vi "SP Format CH Plot.vi"(0 "CH Control":T19={"Trace On"=TRUE, "Measure"=0, "Format"=0, "Autoscale"=TRUE, "Reference"=0.0, "\nRefUnit"="dB/Div", "Position"=5.0, "Scale"=10.0, "ScaleUnit"="dB/Div", "LimitOn"=TRUE, "LimitFill"=FALSE, "Display Data"=0, "Show Markers"=TRUE, "SXX"=""} {"Measure" items=["S11", "S21", "S12", "S22"]; "Reference" format="%#.2g"; "Display Data" items=["Data", "Memory", "Data/Memory"]; "Format" items=["Log Mag", "Phase", "Expanded Phase", "Delay", "Smith", "Polar", "Lin Mag", "SWR", "Loss", "Real", "Imaginary"]; "Scale" min=0.001 step=1.0 format="%#.2g"; "Position" min=0.0 max=10.0}, 1 "Results":waveform(dbl)[](array[waveform]), 2 "Limits":T16[](array[typedef]) {"Parameter"."Stimulus Port" min=1 step=1; "Parameter"."Response Port" min=1 step=1}, 3 "Filter Limits":T1[](array[typedef]) {"Parameter"."Stimulus Port" min=1 step=1; "Parameter"."Response Port" min=1 step=1; "Passband"."Bandwidth Attn" format="%.3g"; "Passband"."Stop/Span" format="%.3g"; "Passband"."Start/Center" format="%.3g"}, 5 "Frequency Attributes":cluster{"F0":dbl, "dF":dbl}, 9 "Formatted Data":bool, 11 "error in (no error)":errorcluster, 12 "Units":T13, 13 "Frequency (MHz) In":cluster{"Start":dbl, "Stop":dbl}) -> (4 "X-Y Plot":cluster{"X":dbl[], "Y":dbl[]}[](array[cluster]), 6 "Frequency (MHz) Out":cluster{"Start":dbl, "Stop":dbl}, 10 "Limit Traces":T15, 15 "error out":errorcluster)   [LabVIEW 2011]
uses:
  TypeDefs/SP Display Trace Controls.ctl
  TypeDefs/SP Display Format.ctl
  TypeDefs/SP Display Data.ctl
  TypeDefs/SP Limit.ctl
  TypeDefs/SP Parameter.ctl
  TypeDefs/SP Format.ctl
  TypeDefs/SP Limit Type.ctl
  TypeDefs/SP Limit Point.ctl
  Test Referential Limit.ctl
  TypeDefs/SP Frequency Units.ctl
  TypeDefs/SP Filter.ctl
  TypeDefs/SP Filter Type.ctl
  TypeDefs/SP Filter Passband.ctl
  TypeDefs/SP Frequency Format.ctl
  TypeDefs/SP Filter Ripple.ctl
  TypeDefs/SP Attenuation Point.ctl
  TypeDefs/SP Attenuation Type.ctl
  TypeDefs/SP Skirt Rejection Point.ctl
  TypeDefs/SP Relative Loss.ctl
panel:
  out "Waveform Plot":cluster{"x0":dbl, "dx":dbl, "Y":dbl[]}[](array[cluster])
  # "Div"
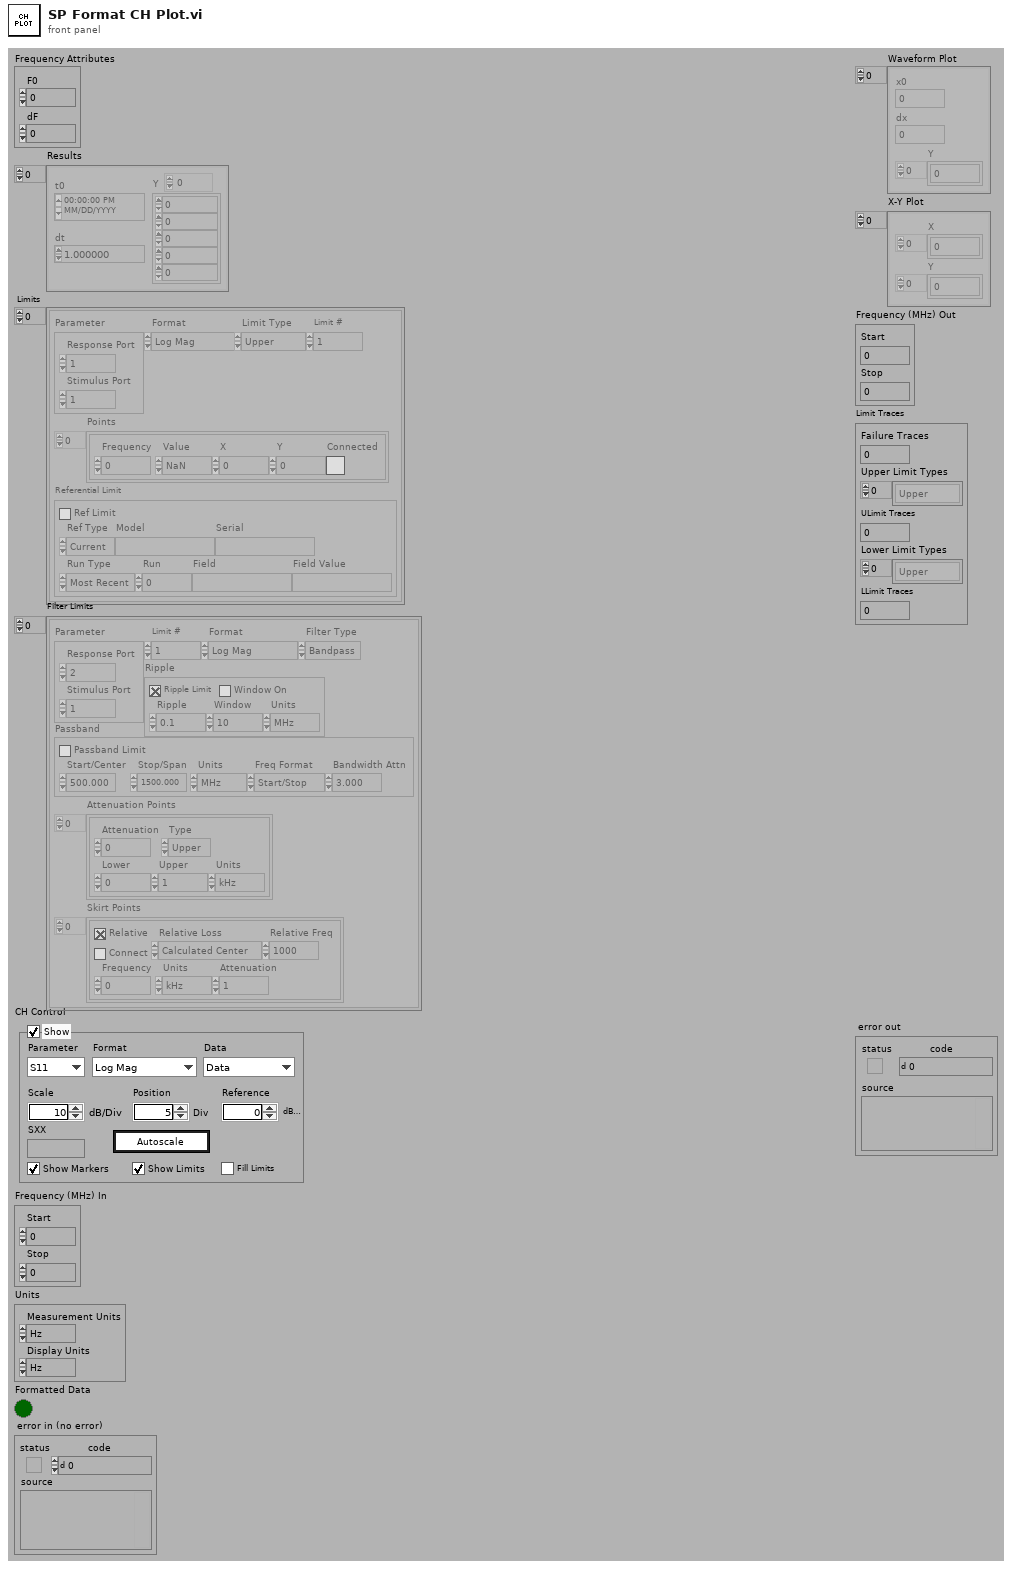
[diagram p1: front panel]
types:
  T1 = typedef "SP Filter.ctl" = cluster{"Limit #":i8, "Parameter":T2, "Format":T3, "Filter Type":T4, "Passband":T5, "Ripple":T8, "Attenuation Points":T9[], "Skirt Points":T11[]}
  T2 = typedef "SP Parameter.ctl" = cluster{"Stimulus Port":i8, "Response Port":i8}
  T3 = typedef "SP Format.ctl" = enum16{"Log Mag", "Lin Mag", "SWR", "Phase", "Expanded Phase", "Delay", "Insertion Loss", "Isolation", "Return Loss"}
  T4 = typedef "SP Filter Type.ctl" = enum16{"Lowpass", "Highpass", "Bandpass", "Bandstop"}
  T5 = typedef "SP Filter Passband.ctl" = cluster{"Start/Center":dbl, "Stop/Span":dbl, "Units":T6, "Freq Format":T7, "Bandwidth Attn":dbl, "Passband Limit":bool}
  T6 = typedef "SP Frequency Units.ctl" = enum16{"Hz", "kHz", "MHz", "GHz", "Points"}
  T7 = typedef "SP Frequency Format.ctl" = enum16{"Start/Stop", "Center/Span"}
  T8 = typedef "SP Filter Ripple.ctl" = cluster{"Ripple Limit":bool, "Window On":bool, "Ripple":dbl, "Window":dbl, "Units":T6}
  T9 = typedef "SP Attenuation Point.ctl" = cluster{"Attenuation":dbl, "Type":T10, "Lower":dbl, "Upper":dbl, "Units":T6}
  T10 = typedef "SP Attenuation Type.ctl" = enum16{"Center", "Lower", "Upper"}
  T11 = typedef "SP Skirt Rejection Point.ctl" = cluster{"Relative":bool, "Connect":bool, "Frequency":dbl, "Units":T6, "Attenuation":dbl, "Relative Loss":T12, "Relative Freq":dbl}
  T12 = typedef "SP Relative Loss.ctl" = enum16{"Calculated Center", "Passband Minimum", "Passband Maximum", "Passband Average", "Frequency"}
  T13 = cluster{"Measurement Units":T6, "Display Units":T6}
  T14 = typedef "SP Limit Type.ctl" = enum16{"Upper", "Lower", "Delta", "Filter", "Referential"}
  T15 = cluster{"Failure Traces":i32, "Upper Limit Types":T14[], "ULimit Traces":i32, "Lower Limit Types":T14[], "LLimit Traces":i32}
  T16 = typedef "SP Limit.ctl" = cluster{"Parameter":T2, "Format":T3, "Limit Type":T14, "Points":T17[], "Referential Limit":T18, "Limit #":i8}
  T17 = typedef "SP Limit Point.ctl" = cluster{"Frequency":dbl, "Value":dbl, "X":dbl, "Y":dbl, "Connected":bool}
  T18 = typedef "Test Referential Limit.ctl" = cluster{"Ref Limit":bool, "Ref Type":enum16{"Current", "Specify"}, "Model":string, "Serial":string, "Run Type":enum16{"Most Recent", "Run #", "Match Field"}, "Run":i32, "Field":string, "Field Value":string}
  T19 = typedef "SP Display Trace Controls.ctl" = cluster{"Trace On":bool, "Measure":i32, "Format":T20, "Autoscale":bool, "Reference":dbl, "\nRefUnit":string, "Position":dbl, "Scale":dbl, "ScaleUnit":string, "LimitOn":bool, "LimitFill":bool, "Display Data":T21, "Show Markers":bool, "SXX":string}
  T20 = typedef "SP Display Format.ctl" = i32
  T21 = typedef "SP Display Data.ctl" = u16
  T22 = cluster{"F0":dbl, "dF":dbl, "Formatted Values":dbl[]}
  T23 = cluster{"F0":dbl, "dF":dbl, "Formatted Values":dbl[]}[]
  T24 = cluster{"Waveform Names[0]":string, "Waveform Names[1]":string, "Waveform Names[2]":string}
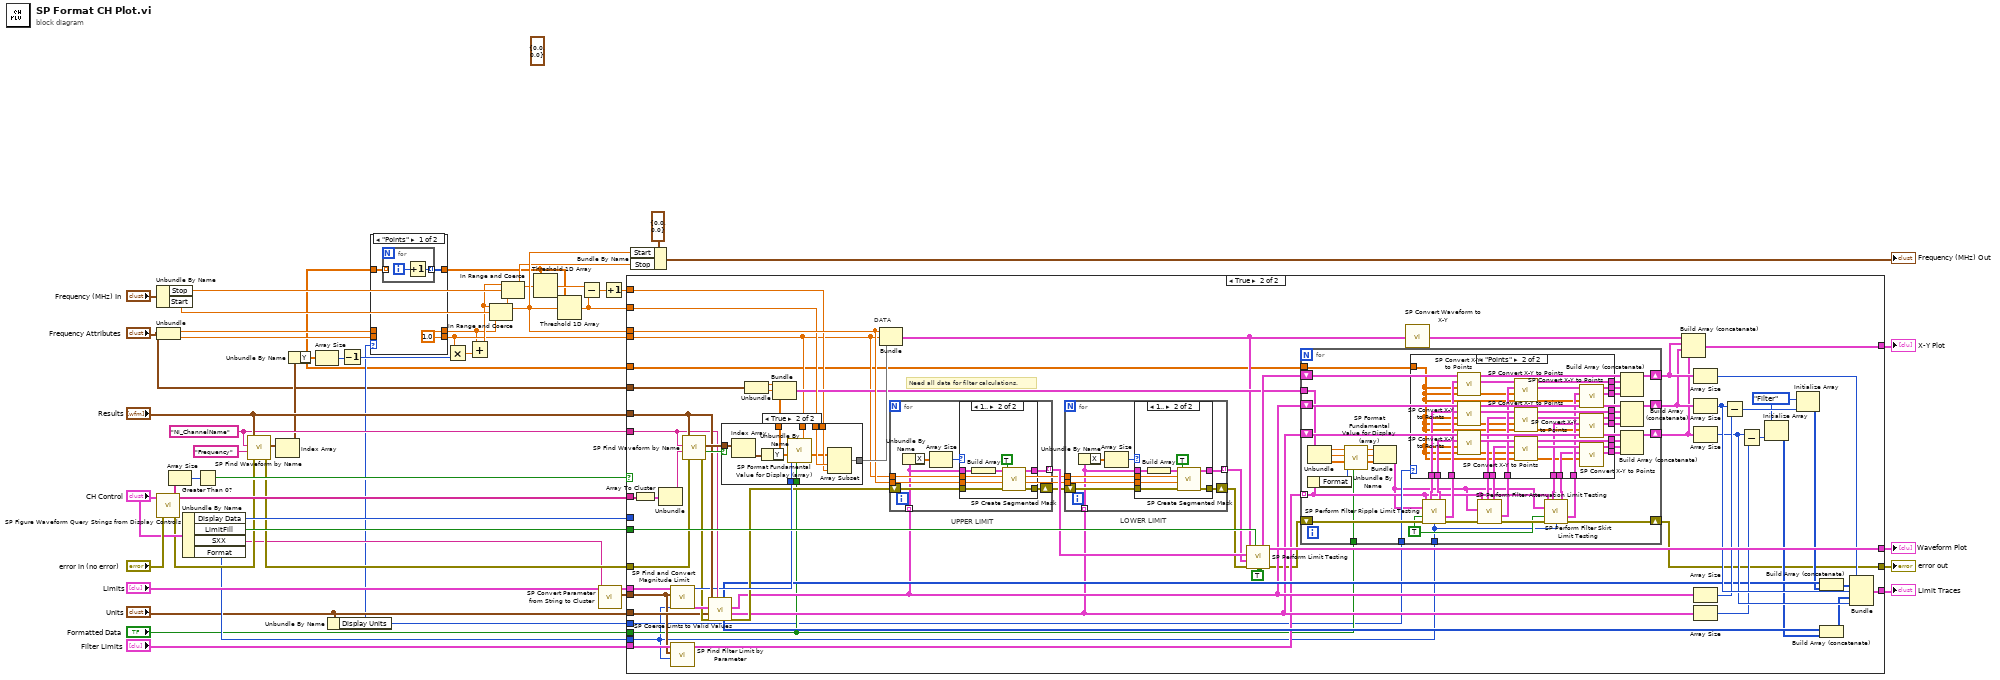
[diagram p0: block diagram]
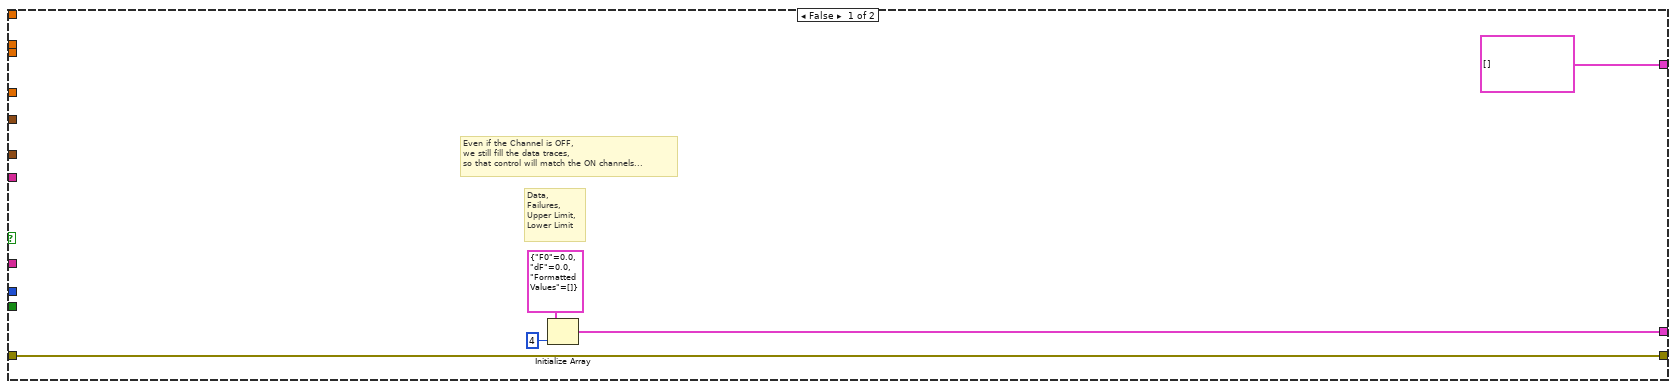
[diagram p3: hidden frame]
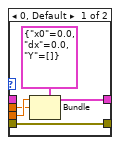
[diagram p5: hidden frame]
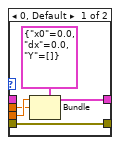
[diagram p6: hidden frame]
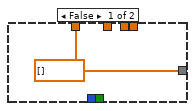
[diagram p7: hidden frame]
diagram:
  (unwired) cluster{"Start":dbl, "Stop":dbl} {"Start"=0.0, "Stop"=0.0} ("output cluster")
  w38 = "NI_ChannelName" ("Attribute Name (NI_ChannelName)")
  n1 = call "SP Figure Waveform Query Strings from Display Controls.vi"("error in (no error)"="error in (no error)", "CH Control"="CH Control") -> ("error out"=w37:errorcluster, "Waveform Names"=w42:string[])  [unwired: 4 out]
  n2 = Unbundle By Name("Frequency (MHz) In") -> ("Stop"=w20:dbl, "Start"=w19:dbl)
  n3 = Unbundle("Frequency Attributes") -> ("F0"=w10:dbl, "dF"=w9:dbl)
  n4 = Array Size(array=w42) -> (size(s)=w43:i32)
  n5 = Unbundle By Name("CH Control") -> ("Display Data"=w46:T21, "LimitFill"=w45:bool, "SXX"=w22:string, "Format"=w29:T20)
  n6 = Greater Than 0?(x=w43) -> (x > 0?=w44:bool)
  n7 = call "SP Find Waveform by Name.vi"("error in (no error)"=w37, "Attribute Value (\"\")"="Frequency" ("Attribute Value (\"\")"), "Attribute Name (NI_ChannelName)"=w38, "Results"="Results") -> ("error out"=w36:errorcluster, "Waveforms"=w27:waveform(dbl)[])  [unwired: 2 out]
  n8 = Index Array(array=w27) -> (element=w26:waveform(dbl))  [unwired: 1 in]
  n9 = Unbundle By Name(w26) -> ("Y"=w1:dbl[])
  n10 = Array Size(array=w1) -> (size(s)=w17:i32)
  n11 = Unbundle By Name("Units") -> ("Display Units"=w3:T6)
  n12 = Decrement(x=w17) -> (x-1=w8:i32)
  n13 = case shown="\"Points\"" w3 {
    tunnel: [w49 w56] -> w5
    tunnel: [w49 w55] -> w11
    tunnel: w10 -> [_ w56]
    tunnel: w9 -> [_ w55]
    tunnel: w1 -> [w51 w54]
    tunnel: [w50 w54] -> w4
    frame "Points" {
      w49 = 1.0 ("dF")
      n14 = for {
        tunnel: w51 -> [_] mode=indexing
        tunnel: [w52] -> w50 mode=indexing
        i -> [w53]
        n15 = Increment(x=w53) -> (x+1=w52:i32)
      }
    }
    frame Default {
    }
  }
  n16 = Multiply(x=w11, y=w8) -> (x*y=w16:dbl)
  n17 = Add(x=w5, y=w16) -> (x+y=w14:dbl)
  n18 = In Range and Coerce(upper limit=w14, x=w19, lower limit=w5) -> (coerced(x)=w30:dbl)  [unwired: 1 out]
  n19 = In Range and Coerce(upper limit=w14, x=w20, lower limit=w30) -> (coerced(x)=w12:dbl)  [unwired: 1 out]
  n20 = Threshold 1D Array(2:w12, 3:w4) -> (0:w15:dbl)  [unwired: 1 out]
  n21 = Threshold 1D Array(2:w30, 3:w4) -> (0:w35:dbl)  [unwired: 1 out]
  n22 = Subtract(x=w15, y=w35) -> (x-y=w13:dbl)
  n23 = call "SP Convert Parameter from String to Cluster.vi"("Parameter String"=w22) -> ("Parameter"=w23:T2)  [unwired: 10 out]
  n24 = Increment(x=w13) -> (x+1=w24:dbl)
  n25 = case shown="True" w44 {
    tunnel: "Results" -> [_ w115]
    tunnel: w38 -> [_ w114]
    tunnel: w11 -> [_ w68]
    tunnel: w36 -> [w61 w117]
    tunnel: [w61 w77] -> w41
    tunnel: w42 -> [_ w125]
    tunnel: [w58 w110] -> w33
    tunnel: w45 -> [_ w118]
    tunnel: w46 -> [_ _]
    tunnel: w24 -> [_ w69]
    tunnel: w30 -> [_ w75]
    tunnel: w35 -> [_ w74]
    tunnel: "Limits" -> [_ w113]
    tunnel: [cluster{"X":dbl[], "Y":dbl[]}[] [] w111] -> w32
    tunnel: w29 -> [_ w62]
    tunnel: "Formatted Data" -> [_ w64]
    tunnel: [_ w108] -> w25
    tunnel: w23 -> [_ w78]
    tunnel: "Units" -> [_ w101]
    tunnel: "Filter Limits" -> [_ w80]
    tunnel: w3 -> [_ w63]
    tunnel: "Frequency Attributes" -> [_ w70]
    tunnel: w1 -> [_ w65]
    frame False {
      # "Data,\nFailures,\nUpper Limit,\nLower Limit"
      # "Even if the Channel is OFF,\nwe still fill the data traces,\nso that control will match the ON channels..."
      n26 = Initialize Array(T22 {"F0"=0.0, "dF"=0.0, "Formatted Values"=[]}, 4 ("dimension size")) -> (w58:T23)
    }
    frame True {
      w81 = SP_Limit_Type."Filter" ("Limit Type")
      # "Need all data for filter calculations."
      # "LOWER LIMIT"
      # "UPPER LIMIT"
      # "DATA"
      n27 = Array To Cluster(array=w125) -> (cluster=w121:T24)
      n28 = Unbundle(w121) -> ("Waveform Names[0]"=w120:string)  [unwired: 2 out]
      n29 = call "SP Find and Convert Magnitude Limit.vi"("Format"=w62, "Parameter"=w78, "Limits"=w113) -> ("Limits"=w112:T16[], "Limit Format"=w109:T3)  [unwired: 3 out]
      n30 = call "SP Find Filter Limit by Parameter.vi"("Display Format"=w62, "Parameter"=w78, "Filter Limits"=w80) -> ("Filter Limits"=w79:T1[])  [unwired: 8 out]
      n31 = call "SP Find Waveform by Name.vi"("error in (no error)"=w117, "Attribute Value (\"\")"=w120, "Attribute Name (NI_ChannelName)"=w114, "Results"=w115) -> ("error out"=w105:errorcluster, "Found Match?"=w122:bool, "Waveforms"=w124:waveform(dbl)[])  [unwired: 1 out]
      n32 = call "SP Coerce Limts to Valid Values.vi"("Attribute Name (NI_ChannelName)"=w114, "error in (no error)"=w105, "Units"=w101, "Limits"=w112, "Results"=w115) -> ("error out"=w104:errorcluster, "Lower Limit Traces"=w84:cluster{"X":dbl[], "Y":dbl[]}[], "Upper Limit Traces"=w85:cluster{"X":dbl[], "Y":dbl[]}[], "Lower Limit Types"=w90:T14[], "Upper Limit Types"=w91:T14[])  [unwired: 2 out]
      n33 = case shown="True" w122 {
        tunnel: w124 -> [_ w242]
        tunnel: w109 -> [_ w247]
        tunnel: [w237 w240] -> w123
        tunnel: w68 -> [_ w246]
        tunnel: w74 -> [_ w245]
        tunnel: w69 -> [_ w244]
        tunnel: w64 -> [_ w243]
        tunnel: [w237 w238] -> w71
        frame False {
          w237 = dbl[] [] ("Formatted Values")
        }
        frame True {
          n34 = Index Array(array=w242) -> (element=w241:waveform(dbl))  [unwired: 1 in]
          n35 = Unbundle By Name(w241) -> ("Y"=w238:dbl[])
          n36 = call "SP Format Fundamental Value for Display (array).vi"("dF, MHz"=w246, "Formatted Data? (F)"=w243, "Display Format"=w247, "Fundamental Values"=w238) -> ("Formatted Values"=w239:dbl[])  [unwired: 7 out]
          n37 = Array Subset(array=w239, index=w245, length=w244) -> (w240:dbl[])
        }
      }
      n38 = Unbundle(w70) -> ("F0"=w67:dbl, "dF"=w66:dbl)
      n39 = Bundle("F0"=w67, "dF"=w66, "Y"=w71) -> (w73:cluster{"F0":dbl, "dF":dbl, "Y":dbl[]})  [unwired: 1 out]
      n40 = Bundle("F0"=w75, "dF"=w68, "Formatted Values"=w123) -> (w72:T22)  [unwired: 1 out]
      n41 = for {
        tunnel: w85 -> [w217] mode=indexing
        tunnel: w68 -> [w220]
        tunnel: w75 -> [w219]
        shift-right: [w222] -> w103
        shift-left: w104 -> [w221]
        tunnel: [w218] -> w107 mode=indexing
        n42 = Unbundle By Name(w217) -> ("X"=w216:dbl[])
        n43 = Array Size(array=w216) -> (size(s)=w223:i32)
        n44 = case shown="1.." w223 {
          tunnel: [w226 w236] -> w218
          tunnel: w221 -> [w228 w235]
          tunnel: [w228 w234] -> w222
          tunnel: w219 -> [w225 w233]
          tunnel: w220 -> [w224 w232]
          tunnel: w217 -> [_ w230]
          frame 0, Default {
            n45 = Bundle(cluster=cluster{"x0":dbl, "dx":dbl, "Y":dbl[]} {"x0"=0.0, "dx"=0.0, "Y"=[]} ("Limit"), "x0"=w225, "dx"=w224) -> (w226:cluster{"x0":dbl, "dx":dbl, "Y":dbl[]})  [unwired: 1 out]
          }
          frame 1.. {
            n46 = Build Array(w230) -> (w229:cluster{"X":dbl[], "Y":dbl[]}[])
            n47 = call "SP Create Segmented Mask.vi"("Reset"=TRUE, "error in"=w235, "x0"=w233, "dx"=w232, "Specification Cluster"=w229) -> ("error out"=w234:errorcluster, "Limit"=w236:cluster{"x0":dbl, "dx":dbl, "Y":dbl[]})  [unwired: 3 out]
          }
        }
      }
      n48 = for {
        tunnel: w84 -> [w196] mode=indexing
        tunnel: w68 -> [w199]
        tunnel: w75 -> [w198]
        shift-right: [w201] -> w100
        shift-left: w103 -> [w200]
        tunnel: [w197] -> w106 mode=indexing
        n49 = Unbundle By Name(w196) -> ("X"=w195:dbl[])
        n50 = Array Size(array=w195) -> (size(s)=w202:i32)
        n51 = case shown="1.." w202 {
          tunnel: [w205 w215] -> w197
          tunnel: w200 -> [w207 w214]
          tunnel: [w207 w213] -> w201
          tunnel: w198 -> [w204 w212]
          tunnel: w199 -> [w203 w211]
          tunnel: w196 -> [_ w209]
          frame 0, Default {
            n52 = Bundle(cluster=cluster{"x0":dbl, "dx":dbl, "Y":dbl[]} {"x0"=0.0, "dx"=0.0, "Y"=[]} ("Limit"), "x0"=w204, "dx"=w203) -> (w205:cluster{"x0":dbl, "dx":dbl, "Y":dbl[]})  [unwired: 1 out]
          }
          frame 1.. {
            n53 = Build Array(w209) -> (w208:cluster{"X":dbl[], "Y":dbl[]}[])
            n54 = call "SP Create Segmented Mask.vi"("Reset"=TRUE, "error in"=w214, "x0"=w212, "dx"=w211, "Specification Cluster"=w208) -> ("error out"=w213:errorcluster, "Limit"=w215:cluster{"x0":dbl, "dx":dbl, "Y":dbl[]})  [unwired: 3 out]
          }
        }
      }
      n55 = call "SP Perform Limit Testing.vi"("Generate Plot Output? (f)"=TRUE, "Filled Limits? (f)"=w118, "error in (no error)"=w100, "LLimits"=w106, "ULimits"=w107, "Data"=w72) -> ("error out"=w76:errorcluster, "Plot Output"=w110:cluster{"x0":dbl, "dx":dbl, "Y":dbl[]}[], "Failures"=w99:cluster{"x values":dbl[], "y values":dbl[]}[])  [unwired: 1 in, 2 out]
      n56 = for {
        shift-right: [w164] -> w77
        shift-left: w76 -> [w157]
        tunnel: w79 -> [w135] mode=indexing
        tunnel: w73 -> [w128]
        shift-right: [w162] -> w82
        shift-left: w84 -> [w163]
        shift-right: [w160] -> w83
        shift-left: w85 -> [w161]
        shift-right: [w158] -> w98
        shift-left: w99 -> [w159]
        tunnel: w65 -> [w136]
        tunnel: w63 -> [w137]
        tunnel: w64 -> [w133]
        tunnel: w62 -> [w126]
        w156 = TRUE
        n57 = Unbundle(w128) -> ("F0"=w129:dbl, "dF"=w130:dbl, "Y"=w132:dbl[])
        n58 = Unbundle By Name(w135) -> ("Format"=w134:T3)
        n59 = call "SP Format Fundamental Value for Display (array).vi"("dF, MHz"=w130, "Formatted Data? (F)"=w133, "Display Format"=w134, "Fundamental Values"=w132) -> ("Formatted Values"=w131:dbl[])  [unwired: 7 out]
        n60 = Bundle("F0"=w129, "dF"=w130, "Formatted Values"=w131) -> (w127:T22)  [unwired: 1 out]
        n61 = call "SP Perform Filter Ripple Limit Testing.vi"("Filter Limit"=w135, "Data"=w127, "Generate Plot Output? (f)"=w156, "error in (no error)"=w157, "Format"=w126) -> ("Upper Limits"=w153:cluster{"x values":dbl[], "y values":dbl[]}[], "Lower Limits"=w151:cluster{"x values":dbl[], "y values":dbl[]}[], "Failures"=w155:cluster{"x values":dbl[], "y values":dbl[]}[], "error out"=w166:errorcluster)  [unwired: 1 in, 6 out]
        n62 = call "SP Perform Filter Attenuation Limit Testing.vi"("error in (no error)"=w166, "Data"=w127, "Filter Limit"=w135) -> ("error out"=w165:errorcluster, "Failures"=w149:cluster{"x values":dbl[], "y values":dbl[]}[], "Lower Limits"=w145:cluster{"x values":dbl[], "y values":dbl[]}[], "Upper Limits"=w147:cluster{"x values":dbl[], "y values":dbl[]}[])  [unwired: 1 in, 4 out]
        n63 = call "SP Perform Filter Skirt Limit Testing.vi"("Filter Limit"=w135, "Data"=w127, "Generate Plot Output? (f)"=w156, "error in (no error)"=w165, "Format"=w126) -> ("Upper Limits"=w139:cluster{"x values":dbl[], "y values":dbl[]}[], "Lower Limits"=w141:cluster{"x values":dbl[], "y values":dbl[]}[], "Failures"=w142:cluster{"x values":dbl[], "y values":dbl[]}[], "error out"=w164:errorcluster)  [unwired: 1 in, 6 out]
        n64 = case shown="\"Points\"" w137 {
          tunnel: w155 -> [w175 w194]
          tunnel: [w175 w193] -> w154
          tunnel: w153 -> [w172 w192]
          tunnel: [w172 w191] -> w152
          tunnel: w151 -> [w167 w190]
          tunnel: [w167 w189] -> w150
          tunnel: w149 -> [w173 w188]
          tunnel: [w173 w187] -> w148
          tunnel: w147 -> [w171 w186]
          tunnel: [w171 w185] -> w146
          tunnel: w145 -> [w168 w184]
          tunnel: [w168 w183] -> w144
          tunnel: [w174 w182] -> w143
          tunnel: w142 -> [w174 w181]
          tunnel: w141 -> [w169 w180]
          tunnel: [w169 w179] -> w140
          tunnel: w139 -> [w170 w178]
          tunnel: [w170 w177] -> w138
          tunnel: w136 -> [_ w176]
          frame Default {
          }
          frame "Points" {
            n65 = call "SP Convert X-Y to Points.vi"("Frequency"=w176, "X-Y"=w194) -> ("X-Y Points"=w193:cluster{"x values":dbl[], "y values":dbl[]}[])  [unwired: 9 out]
            n66 = call "SP Convert X-Y to Points.vi"("Frequency"=w176, "X-Y"=w192) -> ("X-Y Points"=w191:cluster{"x values":dbl[], "y values":dbl[]}[])  [unwired: 9 out]
            n67 = call "SP Convert X-Y to Points.vi"("Frequency"=w176, "X-Y"=w190) -> ("X-Y Points"=w189:cluster{"x values":dbl[], "y values":dbl[]}[])  [unwired: 9 out]
            n68 = call "SP Convert X-Y to Points.vi"("Frequency"=w176, "X-Y"=w188) -> ("X-Y Points"=w187:cluster{"x values":dbl[], "y values":dbl[]}[])  [unwired: 9 out]
            n69 = call "SP Convert X-Y to Points.vi"("Frequency"=w176, "X-Y"=w186) -> ("X-Y Points"=w185:cluster{"x values":dbl[], "y values":dbl[]}[])  [unwired: 9 out]
            n70 = call "SP Convert X-Y to Points.vi"("Frequency"=w176, "X-Y"=w184) -> ("X-Y Points"=w183:cluster{"x values":dbl[], "y values":dbl[]}[])  [unwired: 9 out]
            n71 = call "SP Convert X-Y to Points.vi"("Frequency"=w176, "X-Y"=w181) -> ("X-Y Points"=w182:cluster{"x values":dbl[], "y values":dbl[]}[])  [unwired: 9 out]
            n72 = call "SP Convert X-Y to Points.vi"("Frequency"=w176, "X-Y"=w178) -> ("X-Y Points"=w177:cluster{"x values":dbl[], "y values":dbl[]}[])  [unwired: 9 out]
            n73 = call "SP Convert X-Y to Points.vi"("Frequency"=w176, "X-Y"=w180) -> ("X-Y Points"=w179:cluster{"x values":dbl[], "y values":dbl[]}[])  [unwired: 9 out]
          }
        }
        n74 = Build Array (concatenate)(w159, w154, w148, w143) -> (w158:cluster{"x values":dbl[], "y values":dbl[]}[])
        n75 = Build Array (concatenate)(w161, w152, w146, w138) -> (w160:cluster{"x values":dbl[], "y values":dbl[]}[])
        n76 = Build Array (concatenate)(w163, w150, w144, w140) -> (w162:cluster{"x values":dbl[], "y values":dbl[]}[])
      }
      n77 = call "SP Convert Waveform to X-Y.vi"("Waveform"=w72) -> ("X-Y"=w116:cluster{"X":dbl[], "Y":dbl[]})
      n78 = Build Array (concatenate)(w116, w98, w83, w82) -> (w111:cluster{"X":dbl[], "Y":dbl[]}[])
      n79 = Array Size(array=w98) -> (size(s)=w102:i32)
      n80 = Array Size(array=w83) -> (size(s)=w97:i32)
      n81 = Array Size(array=w82) -> (size(s)=w95:i32)
      n82 = Array Size(array=w85) -> (size(s)=w96:i32)
      n83 = Array Size(array=w84) -> (size(s)=w94:i32)
      n84 = Subtract(x=w97, y=w96) -> (x-y=w92:i32)
      n85 = Subtract(x=w95, y=w94) -> (x-y=w93:i32)
      n86 = Initialize Array(w81, w93) -> (w86:T14[])
      n87 = Initialize Array(w81, w92) -> (w88:T14[])
      n88 = Build Array (concatenate)(w91, w88) -> (w89:T14[])
      n89 = Build Array (concatenate)(w90, w86) -> (w87:T14[])
      n90 = Bundle(w102, w89, w97, w87, w95) -> (w108:cluster{i32, T14[], i32, T14[], i32})  [unwired: 1 out]
    }
  }
  "error out" <- w41
  "Waveform Plot" <- w33
  "X-Y Plot" <- w32
  "Limit Traces" <- w25
  n91 = Bundle By Name(cluster=cluster{"Start":dbl, "Stop":dbl} {"Start"=0.0, "Stop"=0.0} ("output cluster"), "Start"=w30, "Stop"=w12) -> (→"Frequency (MHz) Out":cluster{"Start":dbl, "Stop":dbl})
